vi "Get Car Position Changed Event.vi"(11 "Car Position Changed in":refnum<class "Car Position Changed.lvclass">) -> (1 "Name":string, 3 "Station":string)   [LabVIEW 2016, in "CLD Exam - Car Wash.lvlib" / "Car Position Changed.lvclass"]
uses:
  Car Position Changed.lvclass
  D:/Repos/Stream/software/Mediator/Classes/Message Interface/Message Interface.lvclass
  Car Position Changed.lvclass/Car Position Changed.ctl
  Mediator/Classes/Message Interface/Message Interface.lvclass
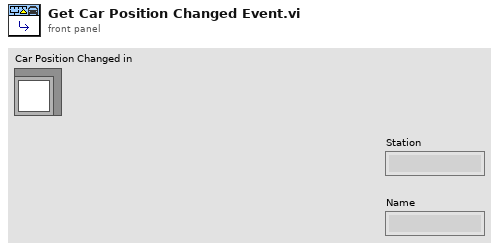
[diagram p1: front panel]
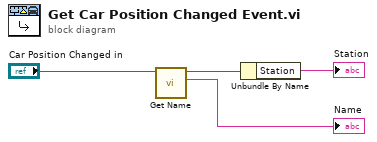
[diagram p0: block diagram]
diagram:
  n1 = call "Get Name.vi"("Message Interface in"="Car Position Changed in") -> ("Name"=→"Name":string, "Message Interface out"=w2:refnum<class "Car Position Changed.lvclass">)  [unwired: 8 in, 1 out]
  n2 = Unbundle By Name(w2) -> ("Station"=→"Station":string)
